vi "ColourCheck.vi"() -> ()   [LabVIEW 2022 SP3]
uses:
  Global Red Initial.vi
  Global Green Initial.vi
  Global Blue Initial.vi
  Output.vi
  Global Red After Box.vi
  Global Green After Box.vi
  Global Blue After Box.vi
panel:
  out "String":string="blue"
  out "String 3":string="red"
  out "String 2":string="green"
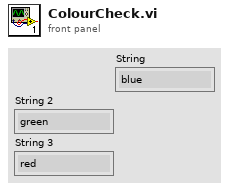
[diagram p1: front panel]
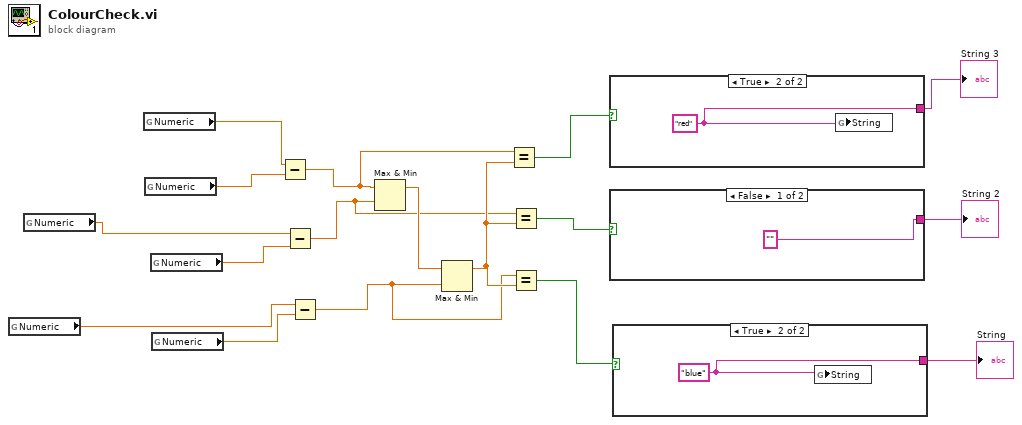
[diagram p0: block diagram]
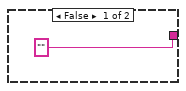
[diagram p2: hidden frame]
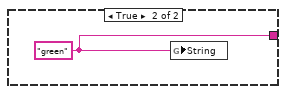
[diagram p3: hidden frame]
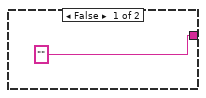
[diagram p4: hidden frame]
diagram:
  n1 = global read "Global Blue After Box.vi" "Numeric"() -> (w1:dbl)
  n2 = global read "Global Green After Box.vi" "Numeric"() -> (w2:dbl)
  n3 = global read "Global Red After Box.vi" "Numeric"() -> (w3:dbl)
  n4 = global read "Global red initial.vi" "Numeric"() -> (w17:dbl)
  n5 = global read "Global green initial.vi" "Numeric"() -> (w16:dbl)
  n6 = global read "Global blue initial.vi" "Numeric"() -> (w15:dbl)
  n7 = Subtract(x=w3, y=w17) -> (x-y=w12:dbl)
  n8 = Subtract(x=w2, y=w16) -> (x-y=w11:dbl)
  n9 = Subtract(x=w1, y=w15) -> (x-y=w10:dbl)
  n10 = Max & Min(x=w12, y=w11) -> (max(x,y)=w14:dbl)  [unwired: 1 out]
  n11 = Max & Min(x=w14, y=w10) -> (max(x,y)=w13:dbl)  [unwired: 1 out]
  n12 = Equal?(x=w12, y=w13) -> (x = y?=w9:bool)
  n13 = Equal?(x=w11, y=w13) -> (x = y?=w8:bool)
  n14 = Equal?(x=w10, y=w13) -> (x = y?=w7:bool)
  n15 = case shown="True" w9 {
    tunnel: ["" w19] -> w5
    frame False {
    }
    frame True {
      w19 = "red"
      n16 = global write "Output.vi" "String"(w19) -> ()
    }
  }
  "String 3" <- w5
  n17 = case shown="False" w8 {
    tunnel: ["" w21] -> w6
    frame False {
    }
    frame True {
      w21 = "green"
      n18 = global write "Output.vi" "String"(w21) -> ()
    }
  }
  "String 2" <- w6
  n19 = case shown="True" w7 {
    tunnel: ["" w23] -> w4
    frame False {
    }
    frame True {
      w23 = "blue"
      n20 = global write "Output.vi" "String"(w23) -> ()
    }
  }
  "String" <- w4
